vi "Line Detector Fit Lorentzian.vi"(6 "Guess":dbl[](array[numeric]), 7 "Frequency":dbl[](array[numeric]), 8 "Error In":errorcluster, 10 "Signal":cdb[](array[numeric]), 11 "Line Detector Configuration":T1={"Peak width guess"=100.0, "Background removal"=enum."NONE", "Smoothing"=enum."NONE", "Smooth window"=100.0, "Relative threshold"=0.0, "Finder algorithm"=enum."Basic", "Bgd window"=100.0, "Spectrum recorder module name"="Spectrum Recorder", "Fit window"=100.0, "Initial fit guess"=enum."Peak finder", "Follow\npeaks"=FALSE, "Re-sample"=nan} {"Re-sample" format="%#_6pHz"; "Fit window" format="%#_6pHz"; "Bgd window" format="%#_6pHz"; "Smooth window" format="%#_6pHz"; "Peak width guess" format="%#_6pHz"}) -> (0 "Error Out":errorcluster, 2 "Plot":cluster{"X":dbl[], "Array":dbl[]}[](array[cluster]), 3 "best fit parameters":dbl[](array[numeric]))   [LabVIEW 2016]
uses:
  LabActor/Post-Processors/Line Detector/Line Detector Configuration.ctl
panel:
  # "F0\n\nAmpl\n\nWidth"
  # "Peak finder config"
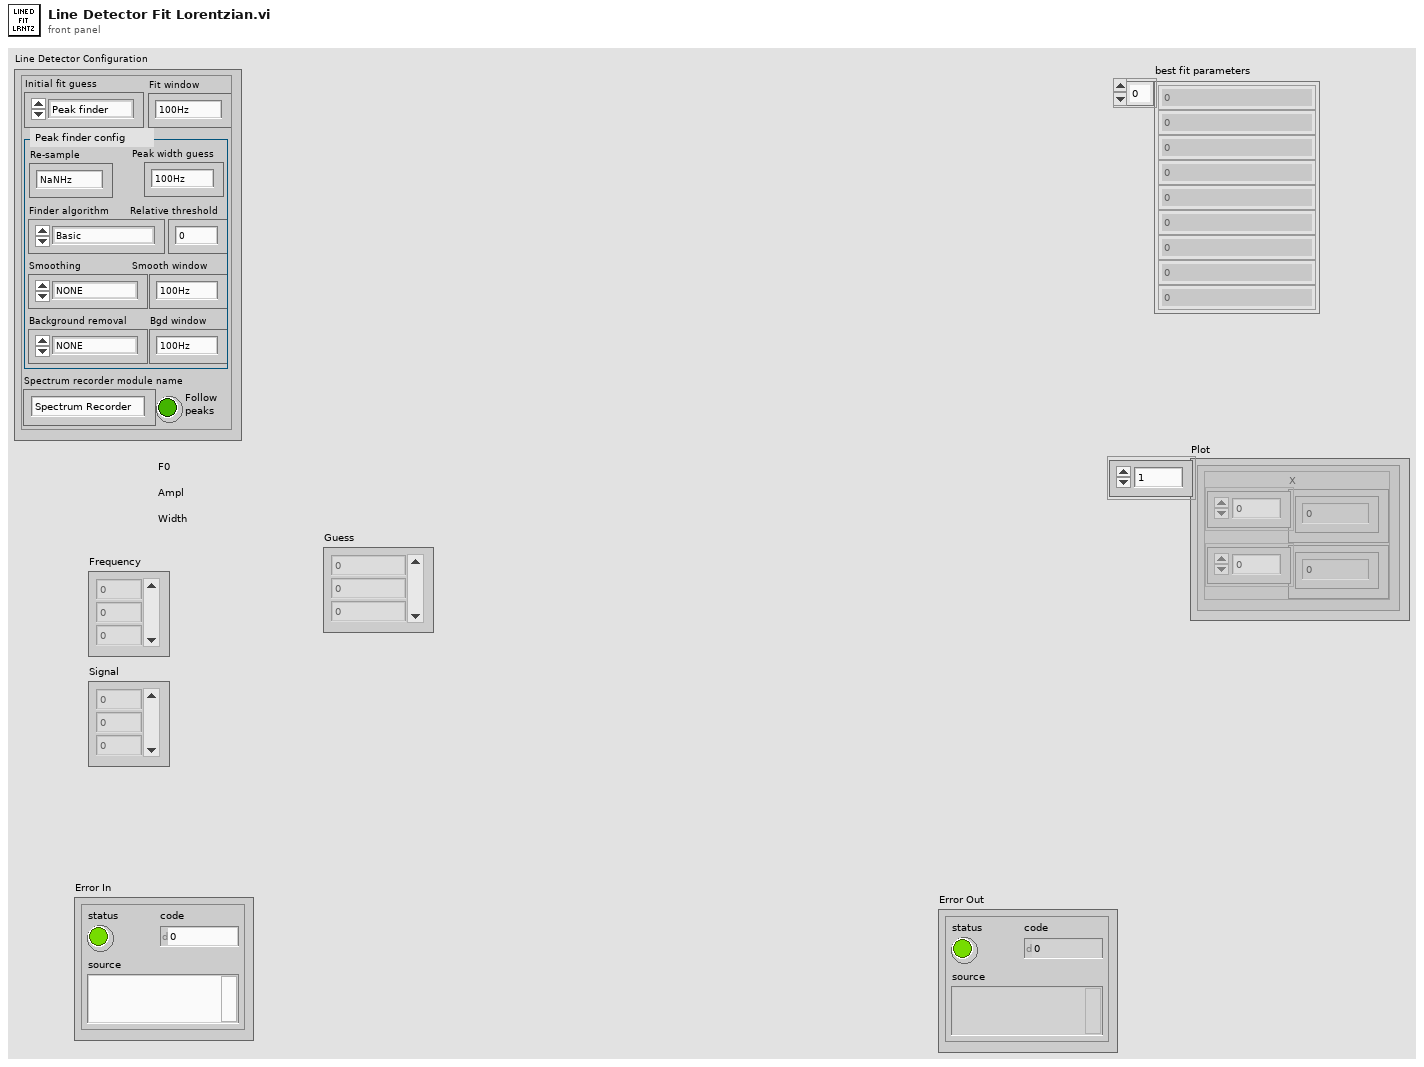
[diagram p1: front panel]
types:
  T1 = typedef "Line Detector Configuration.ctl" = cluster{"Peak width guess":dbl, "Background removal":enum16{"NONE", "High-pass", "Detrend"}, "Smoothing":enum16{"NONE", "Low-pass", "Denoise"}, "Smooth window":dbl, "Relative threshold":dbl, "Finder algorithm":enum16{"Basic", "Wavelet", "Wavelet+detrend"}, "Bgd window":dbl, "Spectrum recorder module name":string, "Fit window":dbl, "Initial fit guess":enum16{"Peak finder", "Last fit"}, "Follow\npeaks":bool, "Re-sample":dbl}
  T2 = cluster{"parameter minimum":dbl[], "parameter maximum":dbl[]}
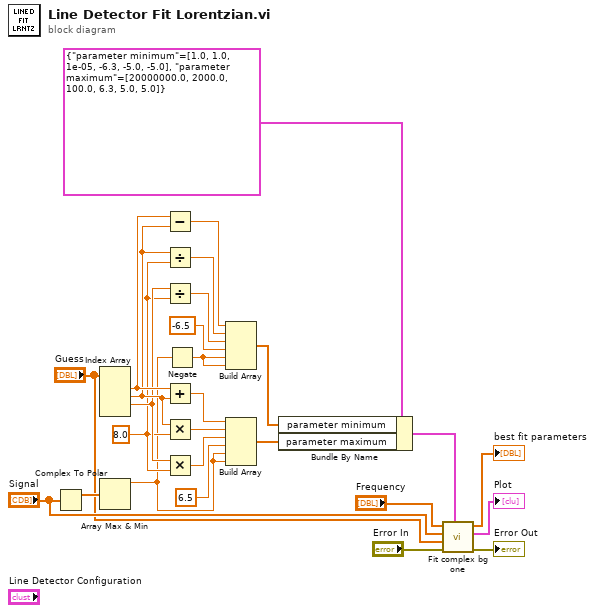
[diagram p0: block diagram]
diagram:
  w8 = 8.0
  n1 = Complex To Polar(r * e^(i*theta)="Signal") -> (r=w3:dbl[])  [unwired: 1 out]
  n2 = Index Array(array="Guess") -> (element #1=w21:dbl, element #2=w19:dbl, element #3=w11:dbl)  [unwired: 4 in, 1 out]
  n3 = Array Max & Min(array=w3) -> (max value=w2:dbl)  [unwired: 3 out]
  n4 = Subtract(x=w21, y=w19) -> (x-y=w22:dbl)
  n5 = Divide(x=w19, y=w8) -> (x/y=w7:dbl)
  n6 = Divide(x=w11, y=w8) -> (x/y=w12:dbl)
  n7 = Add(x=w21, y=w19) -> (x+y=w20:dbl)
  n8 = Multiply(x=w19, y=w8) -> (x*y=w18:dbl)
  n9 = Multiply(x=w11, y=w8) -> (x*y=w10:dbl)
  n10 = Negate(x=w2) -> (-x=w15:dbl)
  n11 = Build Array(w22, w7, w12, -6.5 ("element"), w15, w15) -> (w17:dbl[])
  n12 = Build Array(w20, w18, w10, 6.5 ("element"), w2, w2) -> (w16:dbl[])
  n13 = Bundle By Name(cluster=T2 {"parameter minimum"=[1.0, 1.0, 1e-05, -6.3, -5.0, -5.0], "parameter maximum"=[20000000.0, 2000.0, 100.0, 6.3, 5.0, 5.0]} ("Bounds"), "parameter minimum"=w17, "parameter maximum"=w16) -> (w23:T2)
  n14 = call "Fit complex bg one.vi"("Bounds"=w23, "Error In"="Error In", "Initial parameters"="Guess", "Z"="Signal", "X"="Frequency") -> ("Error Out"=→"Error Out":errorcluster, "Plot"=→"Plot":cluster{"X":dbl[], "Array":dbl[]}[], "best fit parameters"=→"best fit parameters":dbl[])  [unwired: 4 in]
